vi "Clear.vi"(8 "error in (no error)":errorcluster, 11 "Channel in":refnum<data-value>) -> (0 "error out":errorcluster)   [LabVIEW 2020, in "G-Audio.lvlib" / "Channel.lvclass"]
uses:
  Channel.lvclass
  Mixer/Controls/Mixer Audio Data Type.ctl
  Channel.lvclass/Channel.ctl
  af74a676-d843-4657-8a59-58ff5e7e6b53.vi
  ed9d2e0f-d82d-4d1c-95cc-d8a4bf248a02.vi
  Mixer/Mixer.lvclass
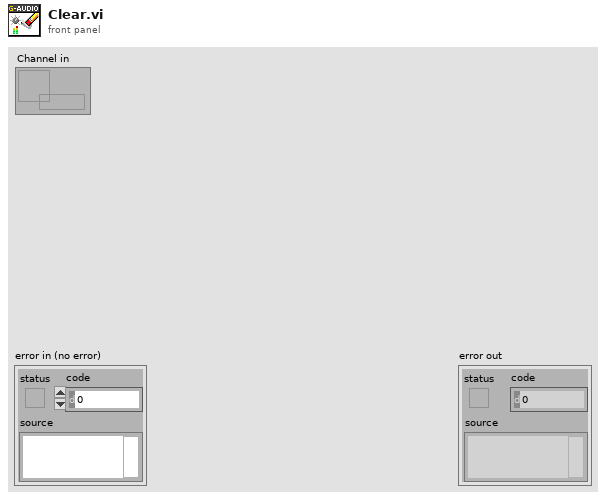
[diagram p1: front panel]
types:
  T1 = typedef "G-Audio.lvlib/Mixer.lvclass/Mixer Audio Data Type.ctl" = i16[][]
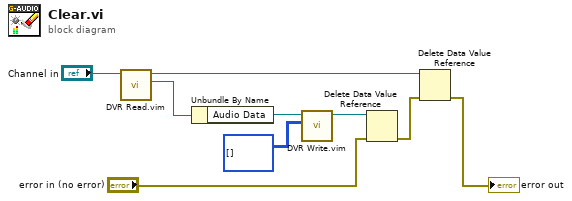
[diagram p0: block diagram]
diagram:
  n1 = call "DVR Read.vim"("DVR In"="Channel in") -> ("Data"=w5:refnum<class "Channel.lvclass">, "DVR Out"=w4:refnum<data-value>)  [unwired: 9 in]
  n2 = Unbundle By Name(w5) -> ("Audio Data"=w9:refnum<data-value>)
  n3 = call "DVR Write.vim"("Data"=T1 [] ("Audio Data Type"), "DVR In"=w9) -> ("DVR Out"=w7:refnum<data-value>)  [unwired: 9 in]
  n4 = Delete Data Value Reference(data value reference=w7, error in="error in (no error)") -> (error out=w3:errorcluster)  [unwired: 1 out]
  n5 = Delete Data Value Reference(data value reference=w4, error in=w3) -> (error out=→"error out":errorcluster)  [unwired: 1 out]
